vi "Motor_control.vi"(0 "Q_in":refnum<queue>, 2 "Param In":T1, 4 "클러스터":T2, 5 "에러 입력(에러 없음)":errorcluster, 6 "문자열":string, 7 "R_force_psd":sgl, 9 "L_force_psd":sgl) -> (14 "Q_out":refnum<queue>, 16 "Param out":T1, 19 "에러 출력":errorcluster)   [LabVIEW 2019]
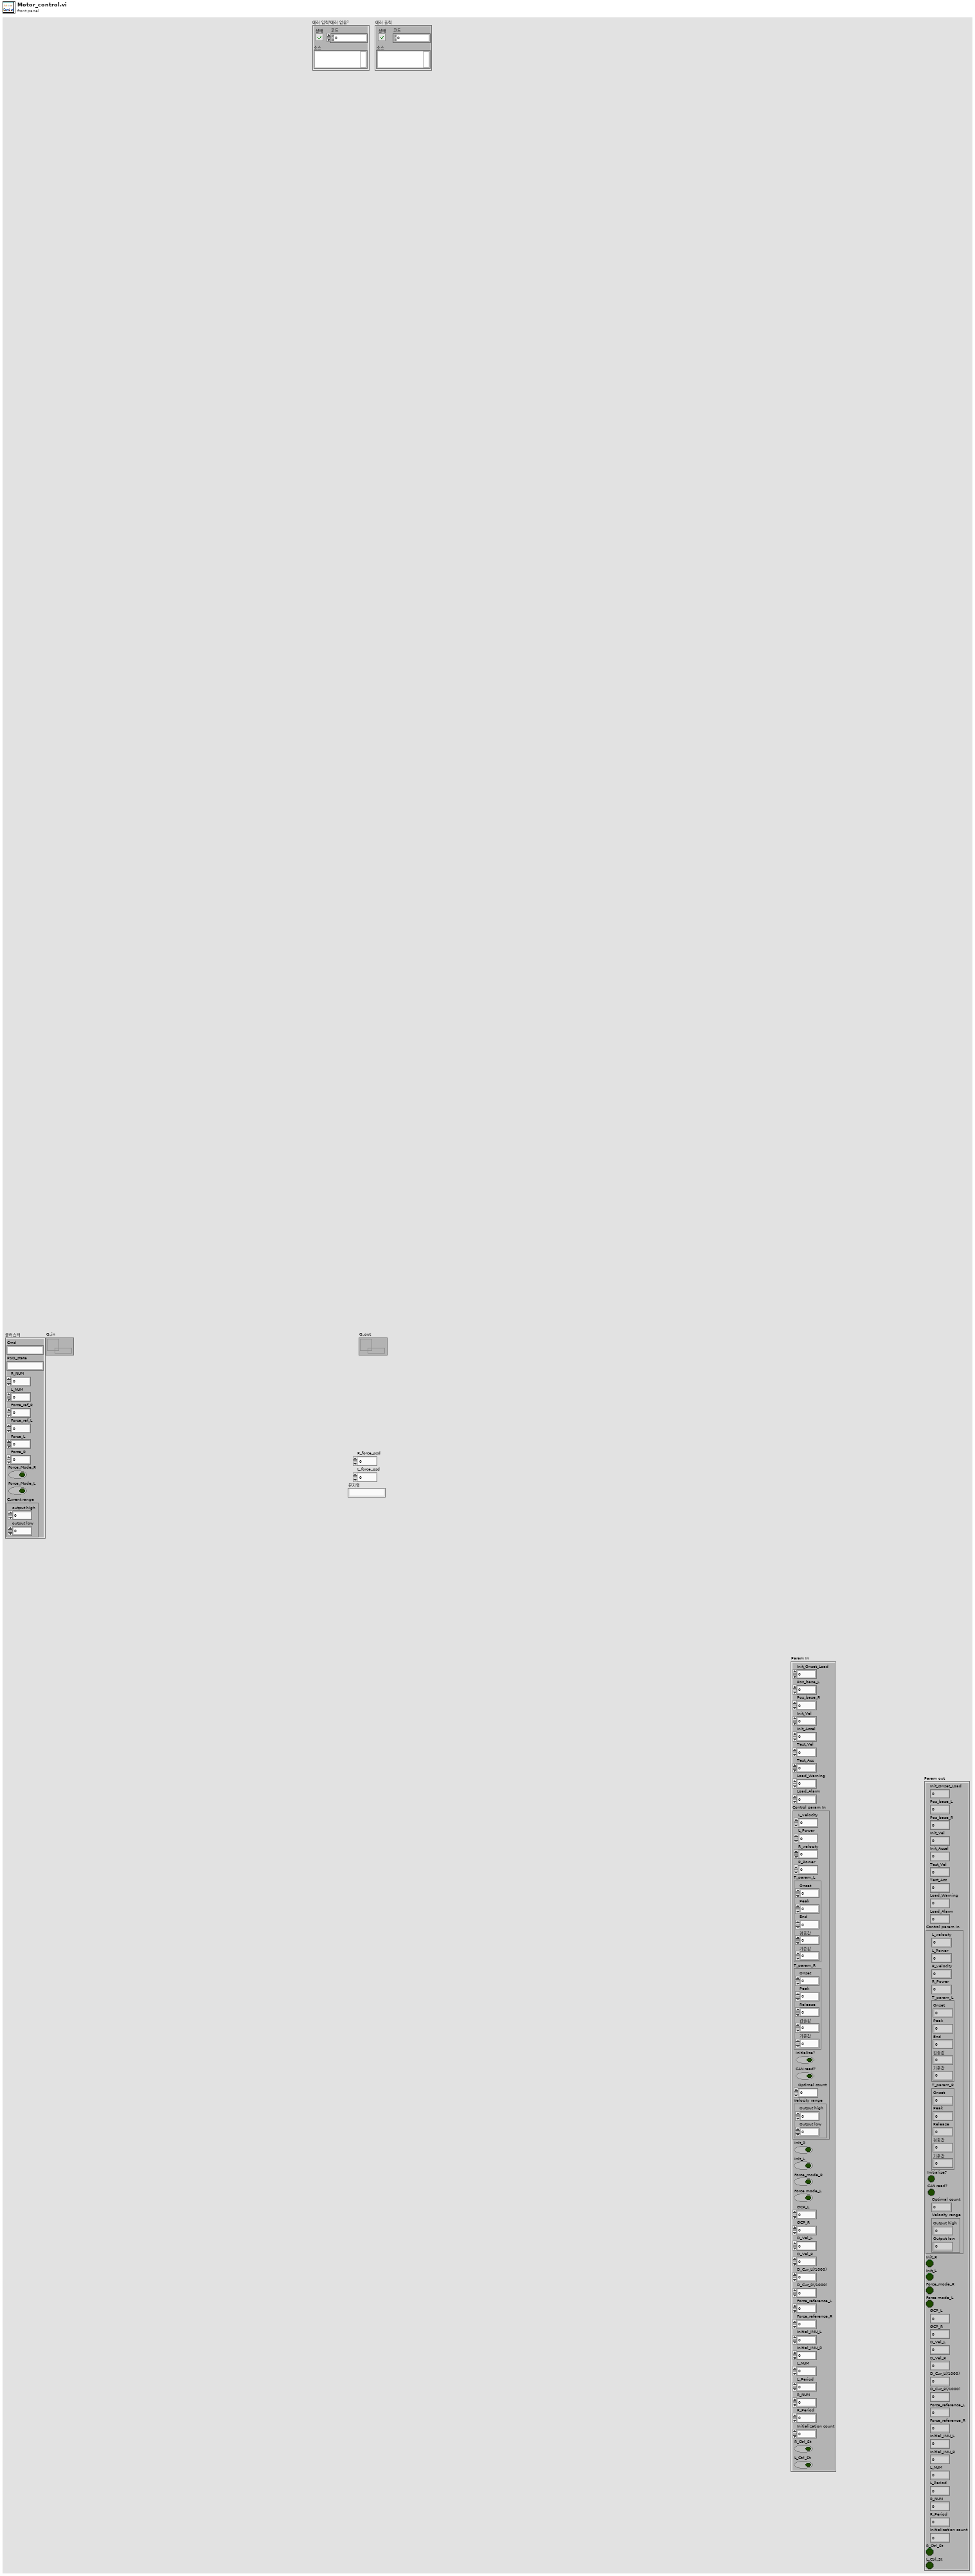
[diagram p1: front panel]
types:
  T1 = cluster{"Init_Onset_Load":sgl, "Pos_base_L":sgl, "Pos_base_R":sgl, "Init_Vel":i32, "Init_Accel":u32, "Test_Vel":i32, "Test_Acc":u32, "Load_Warning":sgl, "Load_Alarm":sgl, "Control param In":cluster{"L_velocity":u32, "L_Power":sgl, "R_velocity":u32, "R_Power":sgl, "T_param_L":cluster{"Onset":sgl, "Peak":sgl, "End":sgl, "검출값":sgl, "기준값":sgl}, "T_param_R":cluster{"Onset":sgl, "Peak":sgl, "Release":sgl, "검출값":sgl, "기준값":sgl}, "Initialize?":bool, "CAN read?":bool, "Optimal count":i32, "Velocity range":cluster{"Output high":dbl, "Output low":dbl}}, "Init_R":bool, "Init_L":bool, "Force_mode_R":bool, "Force mode_L":bool, "GCP_L":sgl, "GCP_R":sgl, "D_Vel_L":sgl, "D_Vel_R":sgl, "D_Cur_L(/1000)":sgl, "D_Cur_R(/1000)":sgl, "Force_reference_L":sgl, "Force_reference_R":sgl, "Initial_IMU_L":sgl, "Initial_IMU_R":sgl, "L_NUM":u32, "L_Period":i16, "R_NUM":u32, "R_Period":i16, "Initialization count":i32, "R_Ctrl_St":bool, "L_Ctrl_St":bool}
  T2 = cluster{"Cmd":string, "PSD_state":string, "R_NUM":u32, "L_NUM":u32, "Force_ref_R":sgl, "Force_ref_L":sgl, "Force_L":sgl, "Force_R":sgl, "Force_Mode_R ":bool, "Force_Mode_L":bool, "Current range":cluster{"output high":dbl, "output low":dbl}}
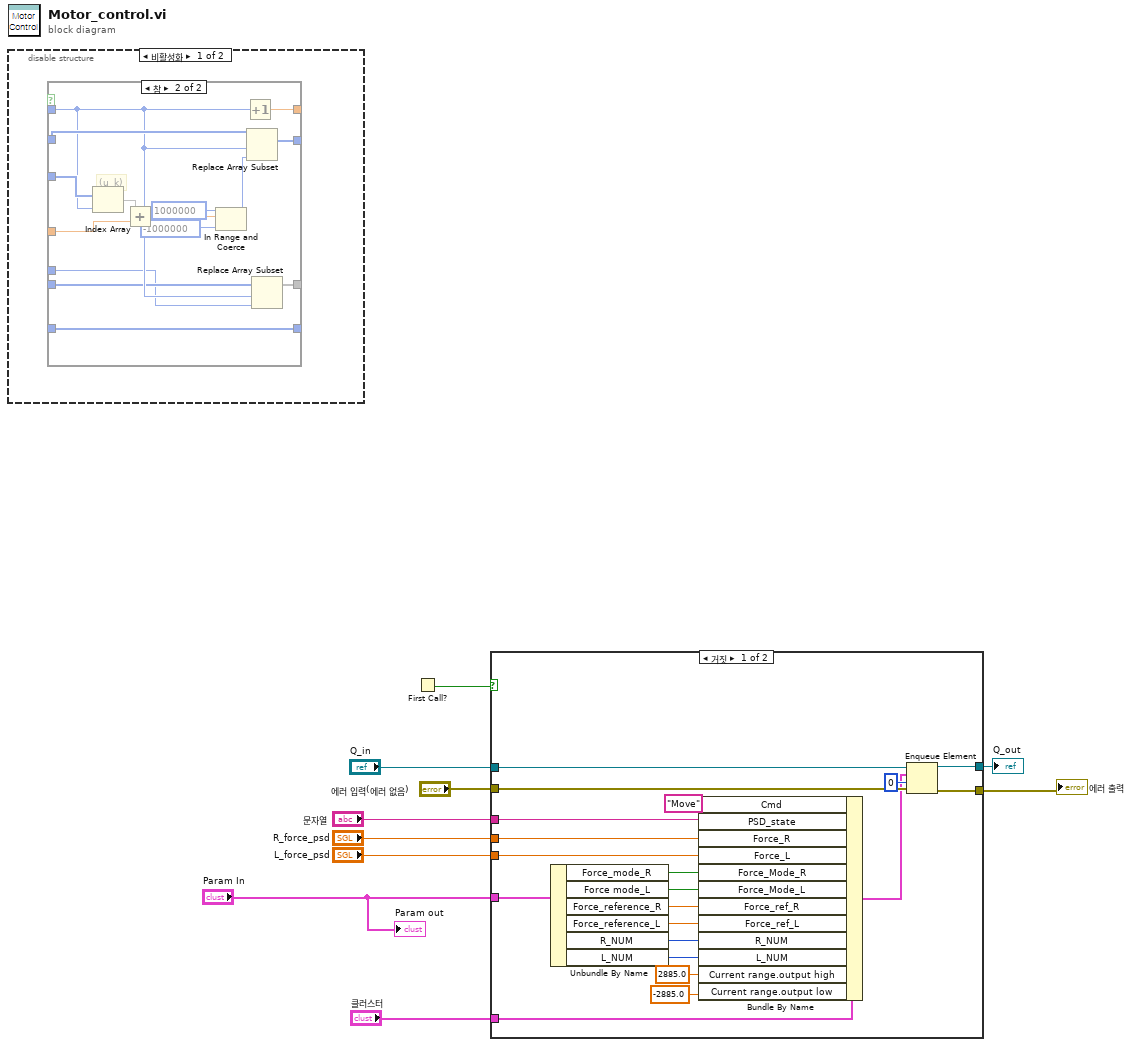
[diagram p0: block diagram]
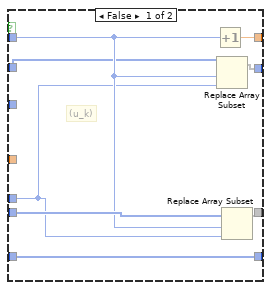
[diagram p2: hidden frame]
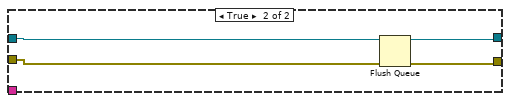
[diagram p4: hidden frame]
diagram:
  n1 = disable-structure shown="비활성화" {
    frame Disabled {
      n2 = case shown="참" {
        selector: _ -> [_ _]
        tunnel: [w13 w33] -> _
        tunnel: _ -> [w12 w32]
        tunnel: [w14 w31] -> _
        tunnel: _ -> [_ w30]
        tunnel: _ -> [_ w28]
        tunnel: _ -> [w15 w27]
        tunnel: _ -> [w18 w26]
        tunnel: [w17 w25] -> _
        tunnel: _ -> [w11 w24]
        tunnel: _ -> [w16 w23]
        tunnel: [w16 w23] -> _
        frame False {
          # "(u_k)"
          n3 = Increment(x=w15) -> (x+1=w14:dbl)
          n4 = Replace Array Subset(array=w12, new element=w11, index=w15) -> (w13:void[])
          n5 = Replace Array Subset(array=w18, new element=w11, index=w15) -> (w17:void[])
        }
        frame True {
          # "(u_k)"
          n6 = Index Array(array=w30, index=w27) -> (element=w29)
          n7 = Add(x=w29, y=w28) -> (x+y=w20:dbl)
          n8 = In Range and Coerce(upper limit=1000000 ("상위 리미트"), x=w20, lower limit=-1000000 ("하위 리미트")) -> (coerced(x)=w19:i32)  [unwired: 1 out]
          n9 = Increment(x=w27) -> (x+1=w31:dbl)
          n10 = Replace Array Subset(array=w32, new element=w19, index=w27) -> (w33:i32[])
          n11 = Replace Array Subset(array=w26, new element=w24, index=w27) -> (w25:void[])
        }
      }
    }
    frame Enabled {
    }
  }
  n12 = First Call?() -> (First Call?: T/F=w8:bool)
  n13 = case shown="거짓" w8 {
    tunnel: "Q_in" -> [w47 w54]
    tunnel: "에러 입력(에러 없음)" -> [w52 w55]
    tunnel: [w51 w57] -> w2
    tunnel: [w50 w56] -> w9
    tunnel: "Param In" -> [w48 _]
    tunnel: "문자열" -> [w36 _]
    tunnel: "클러스터" -> [w46 _]
    tunnel: "R_force_psd" -> [w39 _]
    tunnel: "L_force_psd" -> [w38 _]
    frame False {
      n14 = Unbundle By Name(w48) -> ("Force_mode_R"=w40:bool, "Force mode_L"=w41:bool, "Force_reference_R"=w42:sgl, "Force_reference_L"=w43:sgl, "R_NUM"=w44:u32, "L_NUM"=w45:u32)
      n15 = Bundle By Name(cluster=w46, "Cmd"="Move", "PSD_state"=w36, "Force_R"=w39, "Force_L"=w38, "Force_Mode_R"=w40, "Force_Mode_L"=w41, "Force_ref_R"=w42, "Force_ref_L"=w43, "R_NUM"=w44, "L_NUM"=w45, "Current range.output high"=2885.0, "Current range.output low"=-2885.0) -> (w37:T2)
      n16 = Enqueue Element(queue=w47, element=w37, timeout in ms (-1)=0 ("타임아웃(ms) (-1)"), error in (no error)=w52) -> (queue out=w51:refnum<queue>, error out=w50:errorcluster)  [unwired: 1 out]
    }
    frame True {
      n17 = Flush Queue(queue=w54, error in (no error)=w55) -> (queue out=w57:refnum<queue>, error out=w56:errorcluster)  [unwired: 1 out]
    }
  }
  "에러 출력" <- w9
  "Q_out" <- w2
  "Param out" <- "Param In"
